vi "Get SubNumber.vi"(8 "Error In":errorcluster, 11 "reference in":refnum<class "OD Entry.lvclass">) -> (0 "Error Out":errorcluster, 2 "SubNumber":u8 format="%.0x", 3 "reference out":refnum<class "OD Entry.lvclass">)   [LabVIEW 2019, in "Electronic Datasheet.lvlib" / "OD Entry.lvclass"]
uses:
  OD Entry.lvclass
  OD Entry.lvclass/OD Entry.ctl
  Electronic Datasheet.lvlib
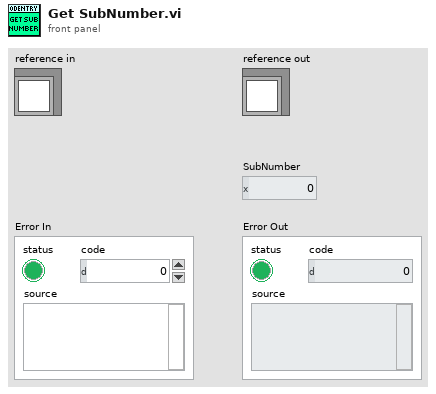
[diagram p1: front panel]
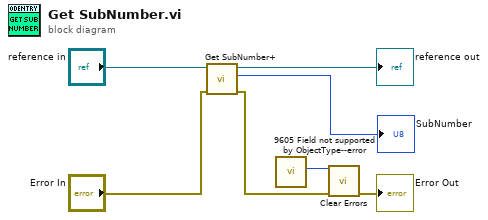
[diagram p0: block diagram]
diagram:
  n1 = call "Get SubNumber+.vi"("Error In"="Error In", "reference in"="reference in") -> ("Error Out"=w4:errorcluster, "SubNumber"=→"SubNumber":u8, "reference out"=→"reference out":refnum<class "OD Entry.lvclass">)  [unwired: 6 in, 1 out]
  n2 = call "9605 Field not supported by ObjectType--error.vi"() -> ("Error Code"=w1:i32)  [unwired: 10 in, 1 out]
  n3 = call <vilib>:"Clear Errors.vi"("error in (no error)"=w4, "specific error code to clear (0: all)"=w1) -> ("error out"=→"Error Out":errorcluster)  [unwired: 4 in, 1 out]
